vi "Calculate Z step size.vi"(9 "Step":dbl, 10 "Stop":dbl, 11 "Start":dbl) -> (1 "AOL Z values":dbl[](array[numeric])=[-200.0, -150.0, -100.0, -50.0, 0.0, 50.0, 100.0, 150.0, 200.0], 2 "Motor Z values":i32[](array[numeric]), 3 "Number of steps":i32)   [LabVIEW 2020]
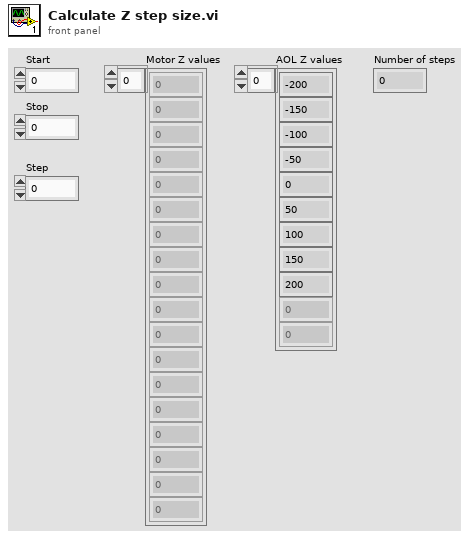
[diagram p1: front panel]
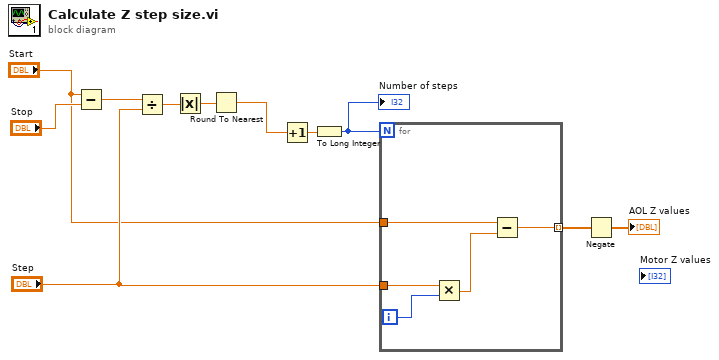
[diagram p0: block diagram]
diagram:
  n1 = Subtract(x="Start", y="Stop") -> (x-y=w9:dbl)
  n2 = Divide(x=w9, y="Step") -> (x/y=w4:dbl)
  n3 = Absolute Value(x=w4) -> (abs(x)=w3:dbl)
  n4 = Round To Nearest(number=w3) -> (nearest integer value=w2:dbl)
  n5 = Increment(x=w2) -> (x+1=w10:dbl)
  n6 = To Long Integer(number=w10) -> (32bit integer=w1:i32)
  "Number of steps" <- w1
  n7 = for {
    N: w1 -> [_]
    tunnel: "Start" -> [w16]
    tunnel: "Step" -> [w15]
    tunnel: [w12] -> w7 mode=indexing
    i -> [w14]
    n8 = Multiply(x=w15, y=w14) -> (x*y=w13:dbl)
    n9 = Subtract(x=w16, y=w13) -> (x-y=w12:dbl)
  }
  n10 = Negate(x=w7) -> (-x=→"AOL Z values":dbl[])
